vi "Reset all slots to empty.vi"(8 "error in":errorcluster, 11 "WorkTable Class in":refnum<class "WorkTable Class.lvclass">) -> (0 "error out":errorcluster, 3 "WorkTable Class out":refnum<class "WorkTable Class.lvclass">)   [LabVIEW 2011, in "WorkTable Class.lvclass"]
uses:
  WorkTable Class.lvclass
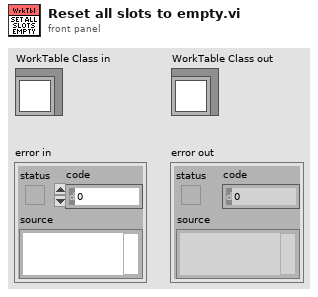
[diagram p1: front panel]
types:
  T1 = enum16{"Empty", "Bare HDI", "Unglued", "Stamped", "PartOnTop", "Weighted", "Unpotted", "Potted"}
  T2 = typedef "Worktable_Stamp.ctl" = cluster{"Stamp State":enum16{"Empty", "Populated", "Used"}, "Location/Orientation":T3, "Stamp Type":T4}
  T3 = typedef "Position_Orientation.ctl" = cluster{"Center":refnum<class "Vec3d Class.lvclass">, "Orientation":refnum<class "Orient3d Class.lvclass">}
  T4 = typedef "Stamp Type.ctl" = enum16{"Stamp 1", "Stamp 2", "Stamp 3", "Stamp 4", "Stamp 5"}
  T5 = cluster{"Reservoir State":enum16{"Empty", "Full", "Used"}, "Center":refnum<class "Vec3d Class.lvclass">}
  T6 = typedef "Worktable_Weight.ctl" = cluster{"Weight State":enum16{"Empty", "Populated"}, "Weight Type":T7, "Location/Orientation":T3}
  T7 = typedef "Weight Type.ctl" = enum16{"Weight 1", "Weight 2", "Weight 3", "Weight 4", "Weight 5", "Weight 6", "Weight 7", "Weight 8"}
  T8 = typedef "Worktable_Module Slot.ctl" = cluster{"Slot State":enum16{"Empty", "Bare HDI", "Unglued", "Stamped", "PartOnTop", "Weighted", "Unpotted", "Potted"}, "BBM Type":enum16{"None", "BBM", "GlassSlide"}, "HDI Type":enum16{"None", "HDI", "Polyimide"}, "Vacuum Channel":u8, "Location/Orientation BBM":T3, "Location/Orientation HDI":T3, "S/N":string}
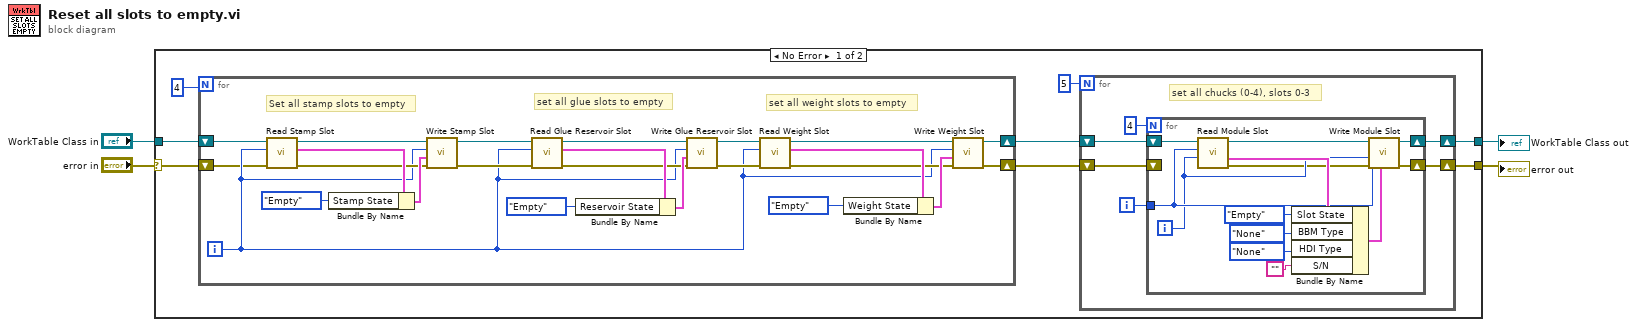
[diagram p0: block diagram]
diagram:
  n1 = case shown="No Error" "error in" {
    selector: "error in" -> [w5 w57]
    tunnel: "WorkTable Class in" -> [w6 w56]
    tunnel: [w8 w56] -> w2
    tunnel: [w7 w57] -> w1
    frame No Error {
      n2 = for {
        N: 4 -> [_]
        shift-right: [w35] -> w9
        shift-left: w5 -> [w32]
        shift-right: [w34] -> w10
        shift-left: w6 -> [w33]
        i -> [w36]
        # "set all weight slots to empty"
        # "set all glue slots to empty"
        # "Set all stamp slots to empty"
        n3 = call "Read Stamp Slot.vi"("error in (no error)"=w32, "Stamp Slot"=w36, "WorkTable Class in"=w33) -> ("error out"=w37:errorcluster, "Stamp Slot"=w55:T2, "WorkTable Class out"=w53:refnum<class "WorkTable Class.lvclass">)  [unwired: 6 in]
        n4 = Bundle By Name(cluster=w55, "Stamp State"=enum16{"Empty", "Populated", "Used"}."Empty") -> (w52:T2)
        n5 = call "Write Stamp Slot.vi"("error in (no error)"=w37, 9:"Stamp Slot"=w52, 10:"Stamp Slot"=w36, "WorkTable Class in"=w53) -> ("error out"=w38:errorcluster, "WorkTable Class out"=w51:refnum<class "WorkTable Class.lvclass">)  [unwired: 6 in]
        n6 = call "Read Glue Reservoir Slot.vi"("error in (no error)"=w38, "index"=w36, "WorkTable Class in"=w51) -> ("error out"=w39:errorcluster, "Glue Resivoir Slot"=w50:T5, "WorkTable Class out"=w48:refnum<class "WorkTable Class.lvclass">)  [unwired: 6 in]
        n7 = Bundle By Name(cluster=w50, "Reservoir State"=enum16{"Empty", "Full", "Used"}."Empty") -> (w47:T5)
        n8 = call "Write Glue Reservoir Slot.vi"("error in (no error)"=w39, "Glue Resivoir Slot"=w47, "index"=w36, "WorkTable Class in"=w48) -> ("error out"=w40:errorcluster, "WorkTable Class out"=w46:refnum<class "WorkTable Class.lvclass">)  [unwired: 6 in]
        n9 = call "Read Weight Slot.vi"("error in (no error)"=w40, "weight slot"=w36, "WorkTable Class in"=w46) -> ("error out"=w41:errorcluster, "Weight Slot"=w44:T6, "WorkTable Class out"=w45:refnum<class "WorkTable Class.lvclass">)  [unwired: 6 in]
        n10 = Bundle By Name(cluster=w44, "Weight State"=enum16{"Empty", "Populated"}."Empty") -> (w42:T6)
        n11 = call "Write Weight Slot.vi"("error in (no error)"=w41, "Weight Slot"=w42, "weight slot"=w36, "WorkTable Class in"=w45) -> ("error out"=w35:errorcluster, "WorkTable Class out"=w34:refnum<class "WorkTable Class.lvclass">)  [unwired: 6 in]
      }
      n12 = for {
        N: 5 -> [_]
        shift-right: [w17] -> w8
        shift-left: w10 -> [w14]
        shift-right: [w16] -> w7
        shift-left: w9 -> [w15]
        i -> [w18]
        # "set all chucks (0-4), slots 0-3"
        n13 = for {
          N: 4 -> [_]
          tunnel: w18 -> [w25]
          shift-right: [w22] -> w17
          shift-left: w14 -> [w31]
          shift-right: [w21] -> w16
          shift-left: w15 -> [_]
          i -> [w24]
          n14 = call-dynamic "Read Module Slot.vi"("slot"=w24, "chuck"=w25, "WorkTable in"=w31) -> ("error out"=w23:errorcluster, "Module Slot"=w29:T8, "WorkTable out"=w30:refnum<class "WorkTable Class.lvclass">)  [unwired: 6 in]
          n15 = Bundle By Name(cluster=w29, "Slot State"=T1."Empty", "BBM Type"=enum16{"None", "BBM", "GlassSlide"}."None", "HDI Type"=enum16{"None", "HDI", "Polyimide"}."None", "S/N"="") -> (w28:T8)
          n16 = call-dynamic "Write Module Slot.vi"("Module Slot"=w28, "error in"=w23, "slot"=w24, "chuck"=w25, "WorkTable in"=w30) -> ("error out"=w21:errorcluster, "WorkTable out"=w22:refnum<class "WorkTable Class.lvclass">)  [unwired: 5 in]
        }
      }
    }
    frame Error {
    }
  }
  "error out" <- w1
  "WorkTable Class out" <- w2
